vi "roboRIO v1.0 Shutdown PWM.vi"(8 "error in (no error)":errorcluster, 10 "Channel":T1, 11 "myRIO Ref In":T2) -> (0 "error out":errorcluster, 3 "myRIO Ref Out":T2)   [LabVIEW 2021]
uses:
  <vilib>/myRIO/Common/Instrument Driver Framework/Utilities/typedefs/myRIO v1.0 Reference.ctl
  <vilib>/myRIO/Common/Instrument Driver Framework/Utilities/typedefs/Generic FPGA Reference.ctl
  <vilib>/myRIO/Common/Instrument Driver Framework/myRIO v1.0/PWM/typedefs/PWM Channels Enum.ctl
  <vilib>/myRIO/Common/Instrument Driver Framework/roboRIO v1.0/PWM/typedefs/roboRIO PWM Channels FPGA Reference.ctl
  <vilib>/rvi/errors/niLvFpgaAdjustHostInterfaceError.vi
  <vilib>/rvi/interface/nirviReadWriteControl/nirviReadWriteControl.xnode
  NiFpgaLv.dll
  <vilib>/rvi/interface/Simulation/niFpgaSimulationCallBeginRW.vi
panel:
  # "This VI turns off the specified PWM channel and zeroes out all of its registers."
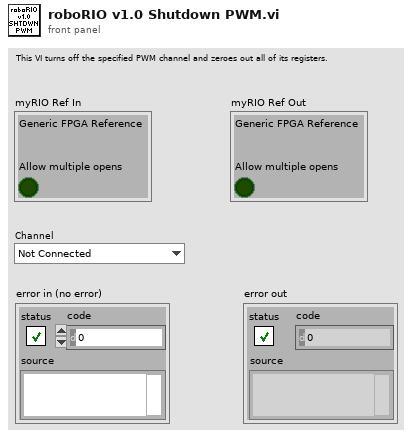
[diagram p1: front panel]
types:
  T1 = typedef "PWM Channels Enum.ctl" = enum16{"Not Connected", "C/PWM0", "C/PWM1", "A/PWM0", "A/PWM1", "A/PWM2", "A/PWM3", "A/PWM4", "A/PWM5", "A/PWM6", "A/PWM7", "A/PWM8", "A/PWM9", "A/PWM10", "A/PWM11", "A/PWM12", "A/PWM13", "A/PWM14", "A/PWM15", "A/PWM16", "A/PWM17", "A/PWM18", "A/PWM19", "B/PWM0", "B/PWM1", "B/PWM2", "B/PWM3", "B/PWM4", "B/PWM5", "B/PWM6", "B/PWM7", "B/PWM8", "B/PWM9", "B/PWM10", "B/PWM11", "B/PWM12", "B/PWM13", "B/PWM14", "B/PWM15", "B/PWM16", "B/PWM17", "B/PWM18", "B/PWM19", "PWM/PWM0", "PWM/PWM1", "PWM/PWM2", "PWM/PWM3", "PWM/PWM4", "PWM/PWM5", "PWM/PWM6", "PWM/PWM7", "PWM/PWM8", "PWM/PWM9"}
  T2 = typedef "myRIO v1.0 Reference.ctl" = cluster{"Generic FPGA Reference":T3, "Allow multiple opens":bool}
  T3 = typedef "Generic FPGA Reference.ctl" = refnum<k20>
  T4 = typedef "roboRIO PWM Channels FPGA Reference.ctl" = refnum<k20>
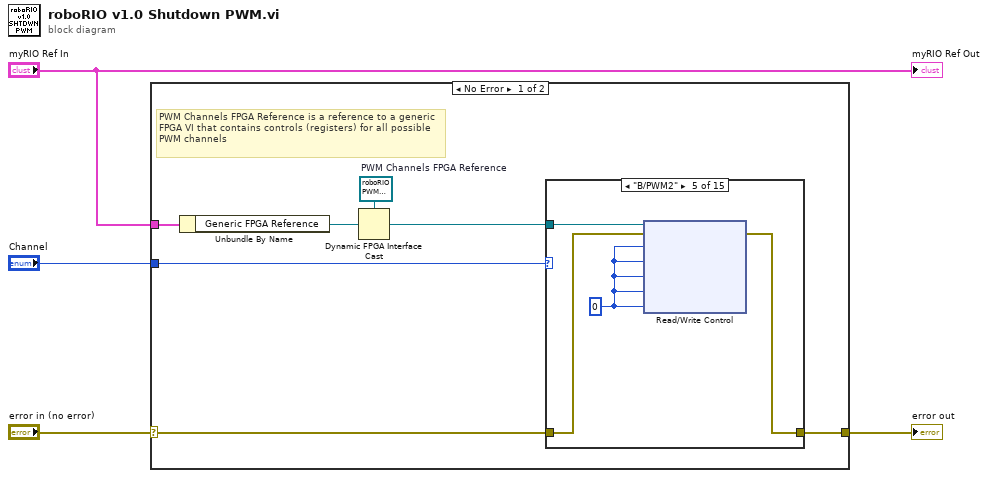
[diagram p0: block diagram]
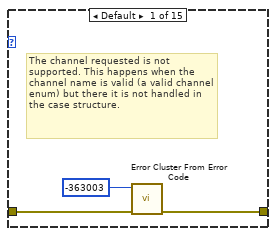
[diagram p2: hidden frame]
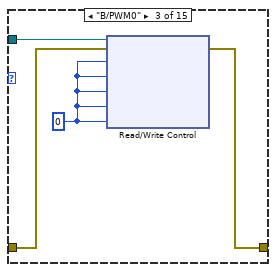
[diagram p4: hidden frame]
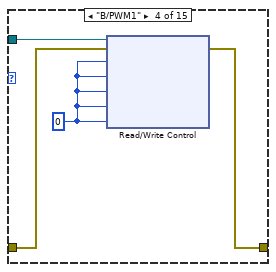
[diagram p5: hidden frame]
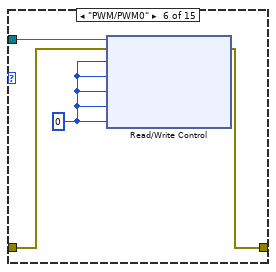
[diagram p6: hidden frame]
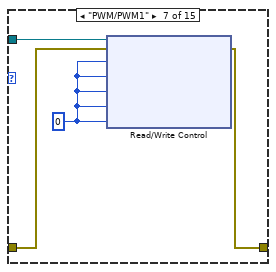
[diagram p7: hidden frame]
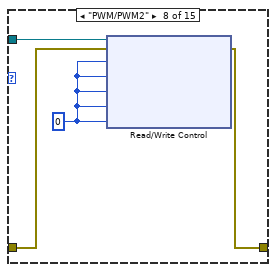
[diagram p8: hidden frame]
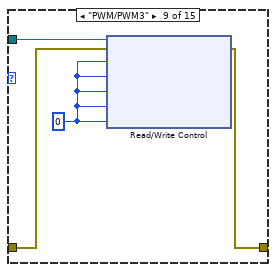
[diagram p9: hidden frame]
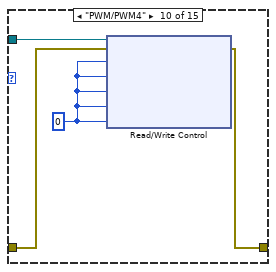
[diagram p10: hidden frame]
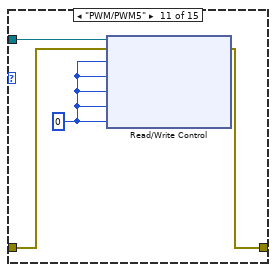
[diagram p11: hidden frame]
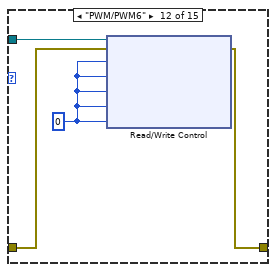
[diagram p12: hidden frame]
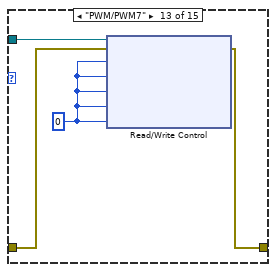
[diagram p13: hidden frame]
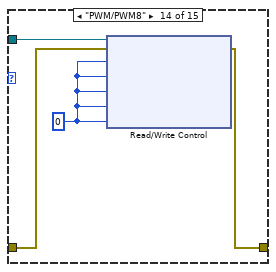
[diagram p14: hidden frame]
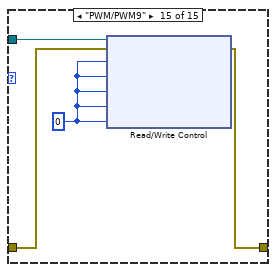
[diagram p15: hidden frame]
diagram:
  n1 = case shown="No Error" "error in (no error)" {
    selector: "error in (no error)" -> [w6 w68]
    tunnel: "myRIO Ref In" -> [w9 _]
    tunnel: [w8 w68] -> w3
    tunnel: "Channel" -> [w7 _]
    frame No Error {
      w11 = T4 refnum  # PWM Channels FPGA Reference
      # "PWM Channels FPGA Reference is a reference to a generic FPGA VI that contains controls (registers) for all possible PWM channels"
      n2 = Unbundle By Name(w9) -> ("Generic FPGA Reference"=w5:T3)
      n3 = Dynamic FPGA Interface Cast(Session In=w11, Type=w5) -> (Session Out=w10:T4)
      n4 = case shown="\"B/PWM2\"" w7 {
        tunnel: w6 -> [w12 w15 w19 w23 w27 w31 w35 w39 w43 w47 w51 w55 w59 w63 w67]
        tunnel: [w13 w15 w18 w22 w26 w30 w34 w38 w42 w46 w50 w54 w58 w62 w66] -> w8
        tunnel: w10 -> [_ _ w17 w21 w25 w29 w33 w37 w41 w45 w49 w53 w57 w61 w65]
        frame Default {
          # "The channel requested is not supported. This happens when the channel name is valid (a valid channel enum) but there it is not handled in the case structure."
          n5 = call <vilib>:"Error Cluster From Error Code.vi"("error in (no error)"=w12, "error code (0)"=-363003) -> ("error out"=w13:errorcluster)  [unwired: 7 in]
        }
        frame "Not Connected" {
        }
        frame "B/PWM0" {
          w16 = u16 0 ("PWM.C_0.MAX")
          n6 = xnode "Read/Write Control"("FPGA VI Reference In"=w17, "error in"=w19, "PWM.B_0.CS"=w16, "PWM.B_0.CNFG"=w16, "PWM.B_0.CNTR"=w16, "PWM.B_0.CMP"=w16, "PWM.B_0.MAX"=w16) -> ("error out"=w18:errorcluster)  [unwired: 1 out]
        }
        frame "B/PWM1" {
          w20 = u16 0 ("PWM.C_0.MAX")
          n7 = xnode "Read/Write Control"("FPGA VI Reference In"=w21, "error in"=w23, "PWM.B_1.CS"=w20, "PWM.B_1.CNFG"=w20, "PWM.B_1.CNTR"=w20, "PWM.B_1.CMP"=w20, "PWM.B_1.MAX"=w20) -> ("error out"=w22:errorcluster)  [unwired: 1 out]
        }
        frame "B/PWM2" {
          w24 = u16 0 ("PWM.C_0.MAX")
          n8 = xnode "Read/Write Control"("FPGA VI Reference In"=w25, "error in"=w27, "PWM.B_2.CS"=w24, "PWM.B_2.CNFG"=w24, "PWM.B_2.CNTR"=w24, "PWM.B_2.CMP"=w24, "PWM.B_2.MAX"=w24) -> ("error out"=w26:errorcluster)  [unwired: 1 out]
        }
        frame "PWM/PWM0" {
          w28 = u16 0 ("PWM.C_0.MAX")
          n9 = xnode "Read/Write Control"("FPGA VI Reference In"=w29, "error in"=w31, "PWM.PWM_0.CS"=w28, "PWM.PWM_0.CNFG"=w28, "PWM.PWM_0.CNTR"=w28, "PWM.PWM_0.CMP"=w28, "PWM.PWM_0.MAX"=w28) -> ("error out"=w30:errorcluster)  [unwired: 1 out]
        }
        frame "PWM/PWM1" {
          w32 = u16 0 ("PWM.C_0.MAX")
          n10 = xnode "Read/Write Control"("FPGA VI Reference In"=w33, "error in"=w35, "PWM.PWM_1.CS"=w32, "PWM.PWM_1.CNFG"=w32, "PWM.PWM_1.CNTR"=w32, "PWM.PWM_1.CMP"=w32, "PWM.PWM_1.MAX"=w32) -> ("error out"=w34:errorcluster)  [unwired: 1 out]
        }
        frame "PWM/PWM2" {
          w36 = u16 0 ("PWM.C_0.MAX")
          n11 = xnode "Read/Write Control"("FPGA VI Reference In"=w37, "error in"=w39, "PWM.PWM_2.CS"=w36, "PWM.PWM_2.CNFG"=w36, "PWM.PWM_2.CNTR"=w36, "PWM.PWM_2.CMP"=w36, "PWM.PWM_2.MAX"=w36) -> ("error out"=w38:errorcluster)  [unwired: 1 out]
        }
        frame "PWM/PWM3" {
          w40 = u16 0 ("PWM.C_0.MAX")
          n12 = xnode "Read/Write Control"("FPGA VI Reference In"=w41, "error in"=w43, "PWM.PWM_3.CS"=w40, "PWM.PWM_3.CNFG"=w40, "PWM.PWM_3.CNTR"=w40, "PWM.PWM_2.CMP"=w40, "PWM.PWM_3.MAX"=w40) -> ("error out"=w42:errorcluster)  [unwired: 1 out]
        }
        frame "PWM/PWM4" {
          w44 = u16 0 ("PWM.C_0.MAX")
          n13 = xnode "Read/Write Control"("FPGA VI Reference In"=w45, "error in"=w47, "PWM.PWM_4.CS"=w44, "PWM.PWM_4.CNFG"=w44, "PWM.PWM_4.CNTR"=w44, "PWM.PWM_4.CMP"=w44, "PWM.PWM_4.MAX"=w44) -> ("error out"=w46:errorcluster)  [unwired: 1 out]
        }
        frame "PWM/PWM5" {
          w48 = u16 0 ("PWM.C_0.MAX")
          n14 = xnode "Read/Write Control"("FPGA VI Reference In"=w49, "error in"=w51, "PWM.PWM_5.CS"=w48, "PWM.PWM_5.CNFG"=w48, "PWM.PWM_5.CNTR"=w48, "PWM.PWM_5.CMP"=w48, "PWM.PWM_5.MAX"=w48) -> ("error out"=w50:errorcluster)  [unwired: 1 out]
        }
        frame "PWM/PWM6" {
          w52 = u16 0 ("PWM.C_0.MAX")
          n15 = xnode "Read/Write Control"("FPGA VI Reference In"=w53, "error in"=w55, "PWM.PWM_6.CS"=w52, "PWM.PWM_6.CNFG"=w52, "PWM.PWM_6.CNTR"=w52, "PWM.PWM_6.CMP"=w52, "PWM.PWM_6.MAX"=w52) -> ("error out"=w54:errorcluster)  [unwired: 1 out]
        }
        frame "PWM/PWM7" {
          w56 = u16 0 ("PWM.C_0.MAX")
          n16 = xnode "Read/Write Control"("FPGA VI Reference In"=w57, "error in"=w59, "PWM.PWM_7.CS"=w56, "PWM.PWM_7.CNFG"=w56, "PWM.PWM_7.CNTR"=w56, "PWM.PWM_7.CMP"=w56, "PWM.PWM_7.MAX"=w56) -> ("error out"=w58:errorcluster)  [unwired: 1 out]
        }
        frame "PWM/PWM8" {
          w60 = u16 0 ("PWM.C_0.MAX")
          n17 = xnode "Read/Write Control"("FPGA VI Reference In"=w61, "error in"=w63, "PWM.PWM_8.CS"=w60, "PWM.PWM_8.CNFG"=w60, "PWM.PWM_8.CNTR"=w60, "PWM.PWM_8.CMP"=w60, "PWM.PWM_8.MAX"=w60) -> ("error out"=w62:errorcluster)  [unwired: 1 out]
        }
        frame "PWM/PWM9" {
          w64 = u16 0 ("PWM.C_0.MAX")
          n18 = xnode "Read/Write Control"("FPGA VI Reference In"=w65, "error in"=w67, "PWM.PWM_9.CS"=w64, "PWM.PWM_9.CNFG"=w64, "PWM.PWM_9.CNTR"=w64, "PWM.PWM_9.CMP"=w64, "PWM.PWM_9.MAX"=w64) -> ("error out"=w66:errorcluster)  [unwired: 1 out]
        }
      }
    }
    frame Error {
      # "Nothing to do since there was an incoming error."
    }
  }
  "error out" <- w3
  "myRIO Ref Out" <- "myRIO Ref In"
